vi "Obtain Request Events.vi"(8 "error in":errorcluster, 10 "Create New? (F)":bool) -> (0 "error out":errorcluster, 2 "Hardware Controller Request Events":T1)   [LabVIEW 2024, in "Hardware Controller.lvlib"]
doc: "This VI Obtains/Creates the Requests events that will be used for other modules to communicate with the module that owns this VI. These Requests events will be accessed only via Public API methods for this module.\n\n<b>NOTE</b>: The contents of this VI are automatically generated and modified by the <b>Tools > DQMH Consortium > DQMH</b> utilities. Consider using those utilities instead of making your own modifications to this VI.\n_____\nBased on DQMH Project Template 7.0.0.1280."
uses:
  Hardware Controller.lvlib
  Request Events--cluster.ctl
  Stop Argument--cluster.ctl
  Show Panel Argument--cluster.ctl
  Hide Panel Argument--cluster.ctl
  Get Module Execution Status Argument--cluster.ctl
  Show Diagram Argument--cluster.ctl
  Start System State Broadcast Helper Loop Argument--cluster.ctl
  Launch EtherCat Argument--cluster.ctl
  Register for Broadcast EtherCAT system state Argument--cluster.ctl
  Launch IOLink Argument--cluster.ctl
  Register for IOLink broadcast Argument--cluster.ctl
  Launch all Hardware Argument--cluster.ctl
  Launch all Hardware (Reply Payload)--cluster.ctl
  Write I16 Argument--cluster.ctl
  Write I16 (Reply Payload)--cluster.ctl
  Write U16 Argument--cluster.ctl
  Write U16 (Reply Payload)--cluster.ctl
  Start EtherCAT Conection Argument--cluster.ctl
  Start EtherCAT Conection (Reply Payload)--cluster.ctl
  Ready Drive Argument--cluster.ctl
  Ready Drive (Reply Payload)--cluster.ctl
  Clear System Fault Argument--cluster.ctl
  Clear System Fault (Reply Payload)--cluster.ctl
  Close EtherCAT Connection Argument--cluster.ctl
  Close EtherCAT Connection (Reply Payload)--cluster.ctl
  Set Error Hardware Controller Argument--cluster.ctl
  Set Error Hardware Controller (Reply Payload)--cluster.ctl
  Start IOLink Connection Argument--cluster.ctl
  Start IOLink Connection (Reply Payload)--cluster.ctl
  Close IOLink Connection Argument--cluster.ctl
  Close IOLink Connection (Reply Payload)--cluster.ctl
  Write Turbine RPM Argument--cluster.ctl
  Write Turbine RPM (Reply Payload)--cluster.ctl
  Write Pump RPM Argument--cluster.ctl
  Write Pump RPM (Reply Payload)--cluster.ctl
  Stop Drives Argument--cluster.ctl
  Stop Drives (Reply Payload)--cluster.ctl
panel:
  # "NOTE: The contents of this VI are automatically generated and modified by the Tools > DQMH Consortium > DQMH utilities. Consider using those utilities instead of making your own modifications to this VI."
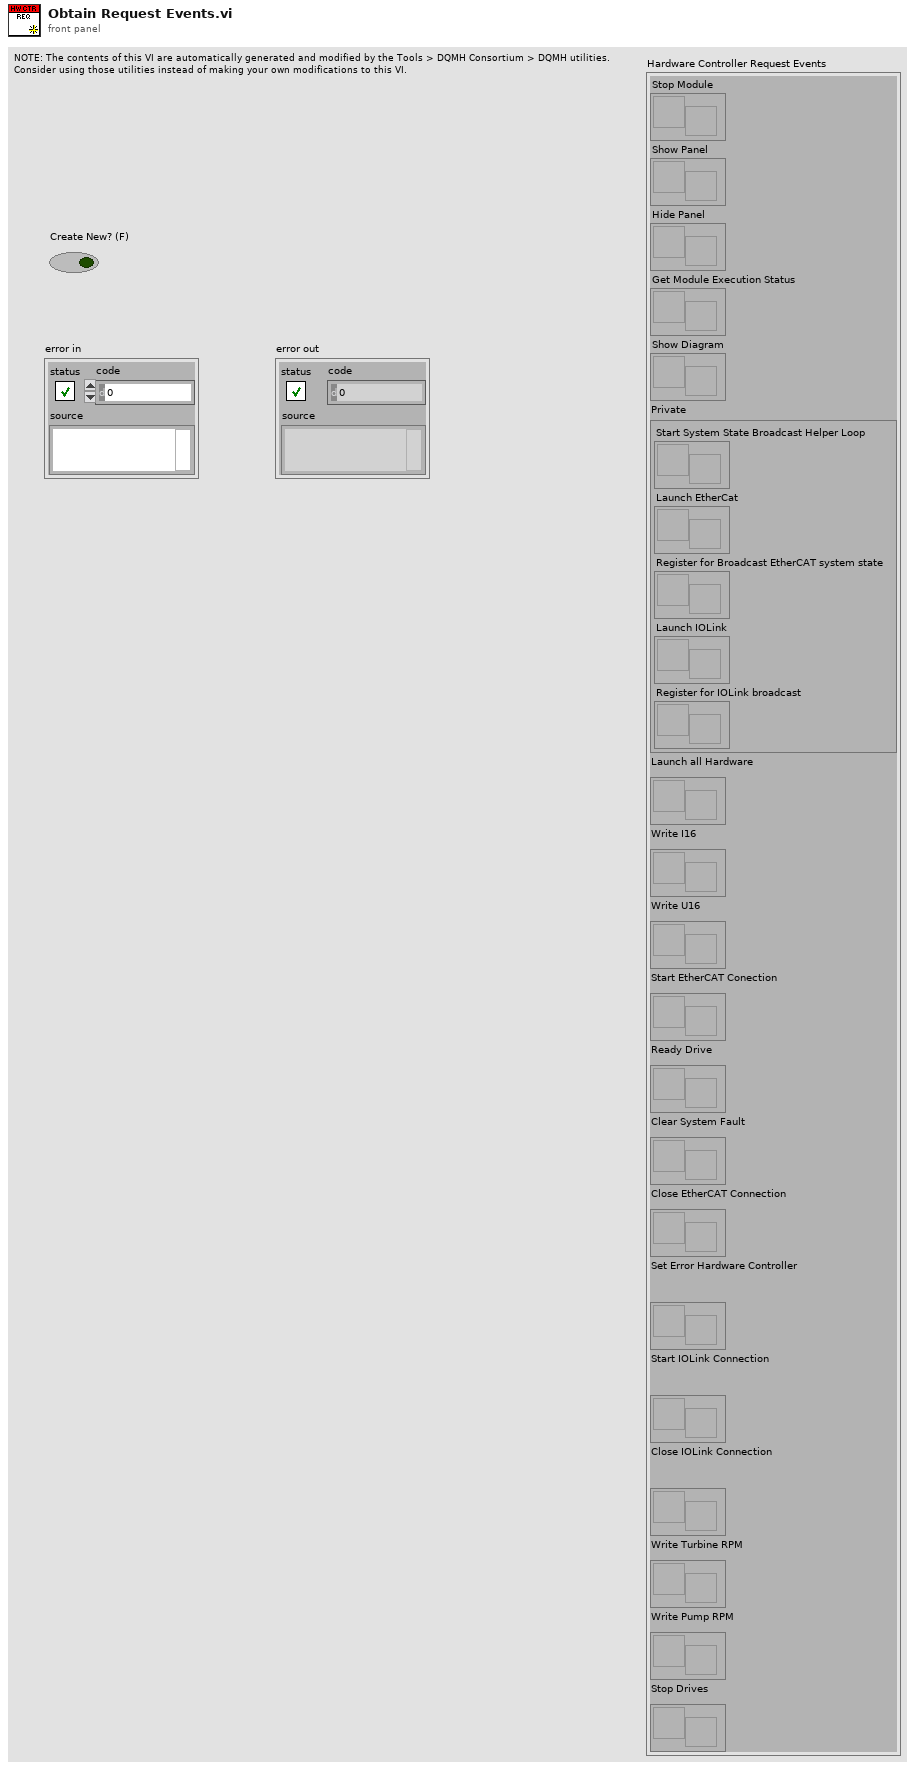
[diagram p1: front panel]
types:
  T1 = typedef "Hardware Controller.lvlib/Request Events--cluster.ctl" = cluster{"Stop Module":refnum<user-event>, "Show Panel":refnum<user-event>, "Hide Panel":refnum<user-event>, "Get Module Execution Status":refnum<user-event>, "Show Diagram":refnum<user-event>, "Private":cluster{"Start System State Broadcast Helper Loop":refnum<user-event>, "Launch EtherCat":refnum<user-event>, "Register for Broadcast EtherCAT system state":refnum<user-event>, "Launch IOLink":refnum<user-event>, "Register for IOLink broadcast":refnum<user-event>}, "Launch all Hardware":refnum<user-event>, "Write I16":refnum<user-event>, "Write U16":refnum<user-event>, "Start EtherCAT Conection":refnum<user-event>, "Ready Drive":refnum<user-event>, "Clear System Fault":refnum<user-event>, "Close EtherCAT Connection":refnum<user-event>, "Set Error Hardware Controller":refnum<user-event>, "Start IOLink Connection":refnum<user-event>, "Close IOLink Connection":refnum<user-event>, "Write Turbine RPM":refnum<user-event>, "Write Pump RPM":refnum<user-event>, "Stop Drives":refnum<user-event>}
  T2 = typedef "Hardware Controller.lvlib/Stop Drives Argument--cluster.ctl" = cluster{"Wait Notifier":refnum<notifier>, "wait for reply":bool}
  T3 = typedef "Hardware Controller.lvlib/Write Pump RPM Argument--cluster.ctl" = cluster{"RPM":i16, "Wait Notifier":refnum<notifier>, "wait for reply":bool}
  T4 = typedef "Hardware Controller.lvlib/Write Turbine RPM Argument--cluster.ctl" = cluster{"RPM":i16, "Wait Notifier":refnum<notifier>, "wait for reply":bool}
  T5 = typedef "Hardware Controller.lvlib/Close IOLink Connection Argument--cluster.ctl" = cluster{"Wait Notifier":refnum<notifier>, "wait for reply":bool}
  T6 = typedef "Hardware Controller.lvlib/Start IOLink Connection Argument--cluster.ctl" = cluster{"Wait Notifier":refnum<notifier>, "wait for reply":bool}
  T7 = typedef "Hardware Controller.lvlib/Set Error Hardware Controller Argument--cluster.ctl" = cluster{"Error Cluster":errorcluster, "Wait Notifier":refnum<notifier>, "wait for reply":bool}
  T8 = typedef "Hardware Controller.lvlib/Register for IOLink broadcast Argument--cluster.ctl" = cluster{"Boolean":bool}
  T9 = typedef "Hardware Controller.lvlib/Launch IOLink Argument--cluster.ctl" = cluster{"Boolean":bool}
  T10 = typedef "Hardware Controller.lvlib/Close EtherCAT Connection Argument--cluster.ctl" = cluster{"Wait Notifier":refnum<notifier>, "wait for reply":bool}
  T11 = typedef "Hardware Controller.lvlib/Clear System Fault Argument--cluster.ctl" = cluster{"Wait Notifier":refnum<notifier>, "wait for reply":bool}
  T12 = typedef "Hardware Controller.lvlib/Ready Drive Argument--cluster.ctl" = cluster{"Drive":string, "Wait Notifier":refnum<notifier>, "wait for reply":bool}
  T13 = typedef "Hardware Controller.lvlib/Start EtherCAT Conection Argument--cluster.ctl" = cluster{"Wait Notifier":refnum<notifier>, "wait for reply":bool}
  T14 = typedef "Hardware Controller.lvlib/Register for Broadcast EtherCAT system state Argument--cluster.ctl" = cluster{"Boolean":bool}
  T15 = typedef "Hardware Controller.lvlib/Write U16 Argument--cluster.ctl" = cluster{"Data":u16, "Drive":string, "Variable":string, "Wait Notifier":refnum<notifier>, "wait for reply":bool}
  T16 = typedef "Hardware Controller.lvlib/Write I16 Argument--cluster.ctl" = cluster{"Drive":string, "Variable":string, "Data":i16, "Wait Notifier":refnum<notifier>, "wait for reply":bool}
  T17 = typedef "Hardware Controller.lvlib/Launch EtherCat Argument--cluster.ctl" = cluster{"Boolean":bool}
  T18 = typedef "Hardware Controller.lvlib/Launch all Hardware Argument--cluster.ctl" = cluster{"Wait Notifier":refnum<notifier>, "wait for reply":bool}
  T19 = typedef "Hardware Controller.lvlib/Start System State Broadcast Helper Loop Argument--cluster.ctl" = cluster{"Boolean":bool}
  T20 = typedef "Hardware Controller.lvlib/Hide Panel Argument--cluster.ctl" = cluster{"Hide Panel?":bool}
  T21 = typedef "Hardware Controller.lvlib/Show Panel Argument--cluster.ctl" = cluster{"Show Panel?":bool}
  T22 = typedef "Hardware Controller.lvlib/Show Diagram Argument--cluster.ctl" = cluster{"Debug?":bool}
  T23 = typedef "Hardware Controller.lvlib/Get Module Execution Status Argument--cluster.ctl" = cluster{"Running?":bool}
  T24 = typedef "Hardware Controller.lvlib/Stop Argument--cluster.ctl" = cluster{"Origin":string, "Exit via Stop Module Req?":bool, "Wait for Module to stop?":bool}
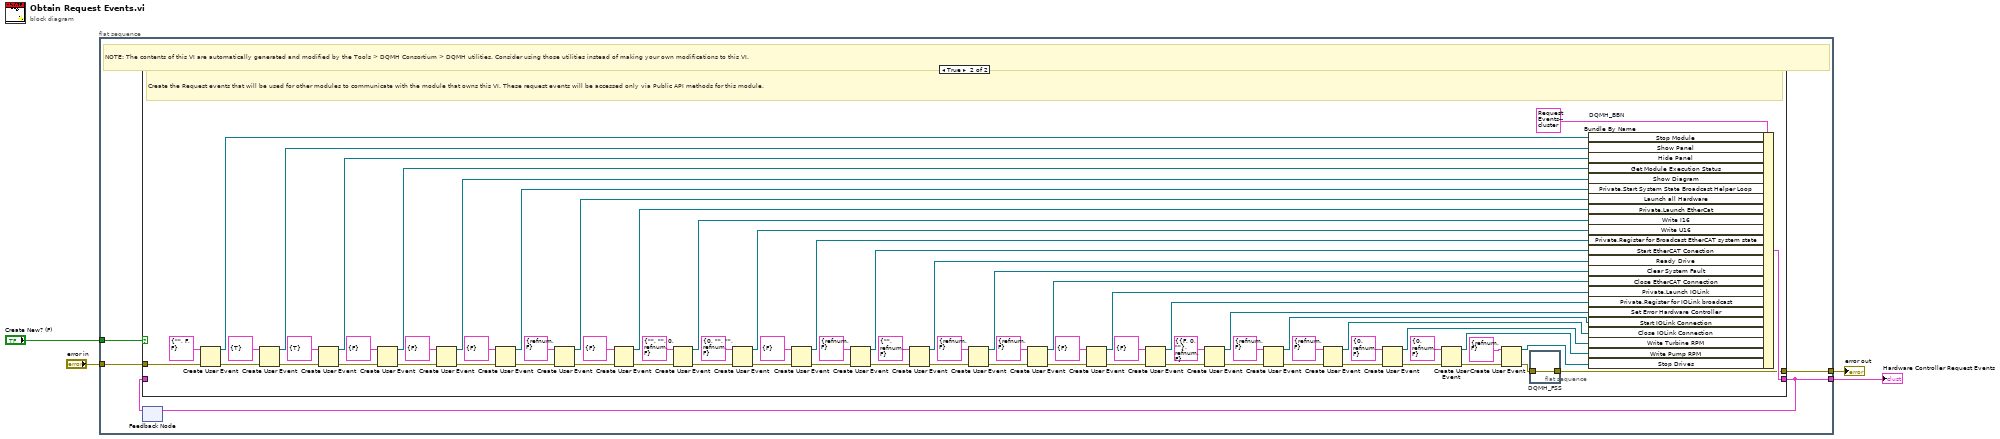
[diagram p0: block diagram]
diagram:
  n1 = flat-sequence {
    tunnel: [w9] -> w4
    tunnel: "error in" -> [w8]
    tunnel: [w6] -> w2
    tunnel: "Create New? (F)" -> [w5]
    frame #0 {
      # "NOTE: The contents of this VI are automatically generated and modified by the Tools > DQMH Consortium > DQMH utilities. Consider using those utilities instead of making your own modifications to this VI."
      n2 = feedback #1() -> (w7:T1)  [unwired: 1 in]
      n3 = case shown="True" w5 {
        tunnel: [w10 w74] -> w9
        tunnel: w8 -> [w10 w84]
        tunnel: [w11 w81] -> w6
        tunnel: w7 -> [w11 _]
        frame False {
          # "Obtain the Request events that were created in a previous call to this VI."
        }
        frame True {
          # "Create the Request events that will be used for other modules to communicate with the module that owns this VI. These request events will be accessed only via Public API methods for this module."
          n4 = Create User Event(user event datatype=T24 {"Origin"="", "Exit via Stop Module Req?"=FALSE, "Wait for Module to stop?"=FALSE} ("Stop Argument"), error in=w84) -> (user event=w82:refnum<user-event>, error out=w79:errorcluster)
          n5 = Create User Event(user event datatype=T21 {"Show Panel?"=TRUE} ("Show Panel Argument"), error in=w79) -> (user event=w78:refnum<user-event>, error out=w77:errorcluster)
          n6 = Create User Event(user event datatype=T20 {"Hide Panel?"=TRUE} ("Hide Panel Argument"), error in=w77) -> (user event=w76:refnum<user-event>, error out=w75:errorcluster)
          n7 = Create User Event(user event datatype=T23 {"Running?"=FALSE} ("Get Module Execution Status Argument"), error in=w75) -> (user event=w72:refnum<user-event>, error out=w73:errorcluster)
          n8 = Create User Event(user event datatype=T22 {"Debug?"=FALSE} ("Show Diagram Argument"), error in=w73) -> (user event=w69:refnum<user-event>, error out=w70:errorcluster)
          n9 = Create User Event(user event datatype=T19 {"Boolean"=FALSE} ("Start System State Broadcast Helper Loop Argument"), error in=w70) -> (user event=w64:refnum<user-event>, error out=w65:errorcluster)
          n10 = Create User Event(user event datatype=T18 {"Wait Notifier"=refnum, "wait for reply"=FALSE} ("Launch all Hardware Argument"), error in=w65) -> (user event=w61:refnum<user-event>, error out=w62:errorcluster)
          n11 = Create User Event(user event datatype=T17 {"Boolean"=FALSE} ("Launch EtherCat Argument"), error in=w62) -> (user event=w58:refnum<user-event>, error out=w59:errorcluster)
          n12 = Create User Event(user event datatype=T16 {"Drive"="", "Variable"="", "Data"=0, "Wait Notifier"=refnum, "wait for reply"=FALSE} ("Write I16 Argument"), error in=w59) -> (user event=w55:refnum<user-event>, error out=w56:errorcluster)
          n13 = Create User Event(user event datatype=T15 {"Data"=0, "Drive"="", "Variable"="", "Wait Notifier"=refnum, "wait for reply"=FALSE} ("Write U16 Argument"), error in=w56) -> (user event=w52:refnum<user-event>, error out=w53:errorcluster)
          n14 = Create User Event(user event datatype=T14 {"Boolean"=FALSE} ("Register for Broadcast EtherCAT system state Argument"), error in=w53) -> (user event=w49:refnum<user-event>, error out=w50:errorcluster)
          n15 = Create User Event(user event datatype=T13 {"Wait Notifier"=refnum, "wait for reply"=FALSE} ("Start EtherCAT Conection Argument"), error in=w50) -> (user event=w46:refnum<user-event>, error out=w47:errorcluster)
          n16 = Create User Event(user event datatype=T12 {"Drive"="", "Wait Notifier"=refnum, "wait for reply"=FALSE} ("Ready Drive Argument"), error in=w47) -> (user event=w43:refnum<user-event>, error out=w44:errorcluster)
          n17 = Create User Event(user event datatype=T11 {"Wait Notifier"=refnum, "wait for reply"=FALSE} ("Clear System Fault Argument"), error in=w44) -> (user event=w40:refnum<user-event>, error out=w41:errorcluster)
          n18 = Create User Event(user event datatype=T10 {"Wait Notifier"=refnum, "wait for reply"=FALSE} ("Close EtherCAT Connection Argument"), error in=w41) -> (user event=w37:refnum<user-event>, error out=w38:errorcluster)
          n19 = Create User Event(user event datatype=T9 {"Boolean"=FALSE} ("Launch IOLink Argument"), error in=w38) -> (user event=w34:refnum<user-event>, error out=w35:errorcluster)
          n20 = Create User Event(user event datatype=T8 {"Boolean"=FALSE} ("Register for IOLink broadcast Argument"), error in=w35) -> (user event=w31:refnum<user-event>, error out=w32:errorcluster)
          n21 = Create User Event(user event datatype=T7 {"Error Cluster"={"status"=FALSE, "code"=0, "source"=""}, "Wait Notifier"=refnum, "wait for reply"=FALSE} ("Set Error Hardware Controller Argument"), error in=w32) -> (user event=w28:refnum<user-event>, error out=w29:errorcluster)
          n22 = Create User Event(user event datatype=T6 {"Wait Notifier"=refnum, "wait for reply"=FALSE} ("Start IOLink Connection Argument"), error in=w29) -> (user event=w25:refnum<user-event>, error out=w26:errorcluster)
          n23 = Create User Event(user event datatype=T5 {"Wait Notifier"=refnum, "wait for reply"=FALSE} ("Close IOLink Connection Argument"), error in=w26) -> (user event=w22:refnum<user-event>, error out=w23:errorcluster)
          n24 = Create User Event(user event datatype=T4 {"RPM"=0, "Wait Notifier"=refnum, "wait for reply"=FALSE} ("Write Turbine RPM Argument"), error in=w23) -> (user event=w19:refnum<user-event>, error out=w20:errorcluster)
          n25 = Create User Event(user event datatype=T3 {"RPM"=0, "Wait Notifier"=refnum, "wait for reply"=FALSE} ("Write Pump RPM Argument"), error in=w20) -> (user event=w16:refnum<user-event>, error out=w17:errorcluster)
          n26 = Create User Event(user event datatype=T2 {"Wait Notifier"=refnum, "wait for reply"=FALSE} ("Stop Drives Argument"), error in=w17) -> (user event=w13:refnum<user-event>, error out=w14:errorcluster)
          n27 = flat-sequence "DQMH_FSS" {
            tunnel: w14 -> [w85]
            tunnel: [w85] -> w74
            frame #0 {
            }
          }
          n28 = Bundle By Name "DQMH_BBN"(cluster=T1 {"Stop Module"=refnum, "Show Panel"=refnum, "Hide Panel"=refnum, "Get Module Execution Status"=refnum, "Show Diagram"=refnum, "Private"={"Start System State Broadcast Helper Loop"=refnum, "Launch EtherCat"=refnum, "Register for Broadcast EtherCAT system state"=refnum, "Launch IOLink"=refnum, "Register for IOLink broadcast"=refnum}, "Launch all Hardware"=refnum, "Write I16"=refnum, "Write U16"=refnum, "Start EtherCAT Conection"=refnum, "Ready Drive"=refnum, "Clear System Fault"=refnum, "Close EtherCAT Connection"=refnum, "Set Error Hardware Controller"=refnum, "Start IOLink Connection"=refnum, "Close IOLink Connection"=refnum, "Write Turbine RPM"=refnum, "Write Pump RPM"=refnum, "Stop Drives"=refnum} ("output cluster"), "Stop Module"=w82, "Show Panel"=w78, "Hide Panel"=w76, "Get Module Execution Status"=w72, "Show Diagram"=w69, "Private.Start System State Broadcast Helper Loop"=w64, "Launch all Hardware"=w61, "Private.Launch EtherCat"=w58, "Write I16"=w55, "Write U16"=w52, "Private.Register for Broadcast EtherCAT system state"=w49, "Start EtherCAT Conection"=w46, "Ready Drive"=w43, "Clear System Fault"=w40, "Close EtherCAT Connection"=w37, "Private.Launch IOLink"=w34, "Private.Register for IOLink broadcast"=w31, "Set Error Hardware Controller"=w28, "Start IOLink Connection"=w25, "Close IOLink Connection"=w22, "Write Turbine RPM"=w19, "Write Pump RPM"=w16, "Stop Drives"=w13) -> (w81:T1)
        }
      }
      n29 = feedback-in #1(w6) -> ()
    }
  }
  "Hardware Controller Request Events" <- w2
  "error out" <- w4
